vi "Sync Reply.vi"(7 "Sender":refnum<class "Sender.lvclass">, 10 "Msg":refnum<class "Msg.lvclass">, 11 "Base Actor in":refnum<class "Base Actor.lvclass">) -> (3 "Base Actor out":refnum<class "Base Actor.lvclass">)   [LabVIEW 2020, in "jettl.lvlib" / "Actor.lvlib" / "Base Actor.lvclass"]
uses:
  Base Actor.lvclass
  Sender/Sender/Sender.lvclass
  Msg/Msg.lvclass
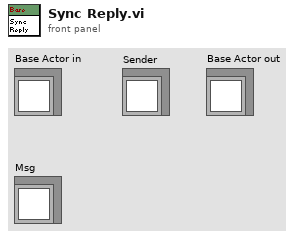
[diagram p1: front panel]
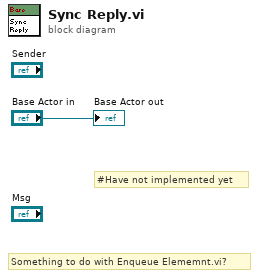
[diagram p0: block diagram]
diagram:
  # "Something to do with Enqueue Elememnt.vi?"
  # "#Have not implemented yet"
  "Base Actor out" <- "Base Actor in"
